vi "Teleop.vi"(10 "Match Info":T1={"Autonomous Elapsed Seconds"=0.0, "TeleOp Elapsed Seconds"=0.0, "Disabled Elapsed Seconds"=0.0, "Visited Autonomous"=FALSE, "Visited TeleOp"=FALSE, "Visited Disabled"=FALSE, "Autonomous Settings"={"Autonomous Style"=enum."Independent", "VI Refnum"=refnum}}, 11 "Call Context":T2) -> ()   [LabVIEW 2015]
doc: "This VI is called for each TeleOp packet received from the DS where the robot is not disabled. It is often used to read from the joysticks and update I/O or to update setpoints for timed control loops. It should complete and return within 20 milliseconds or it may miss DS packets."
uses:
  <vilib>/Rock Robotics/WPI/DriverStation/WPI_DriverStationDerivedRobotMode.ctl
  <vilib>/Rock Robotics/WPI/DriverStation/WPI_DriverStationMatch Info.ctl
  <vilib>/Rock Robotics/Network Tables/NT Read Boolean.vi
  <vilib>/Rock Robotics/Network Tables/NT Read Number.vi
  <vilib>/Rock Robotics/WPI/Utilities/WPI_GetSetVariantRefNum.vi
  <vilib>/Rock Robotics/WPI/RobotDrive/WPI_RobotDriveArcadeDrive_Standard(NoSaturation).vi
  <vilib>/Rock Robotics/Network Tables/NT Write Numeric Array.vi
  Mr. Thayer 2.0.vi
  Mr. Thayer.vi
  <vilib>/Rock Robotics/Network Tables/NT Write Boolean Array.vi
  Global 3.vi
  Global 4.vi
panel:
  out "Sample Slider 0":dbl(slide) scale=0.0..5.0
  out "Sample Boolean 1":bool
  out "Sample Boolean 0":bool
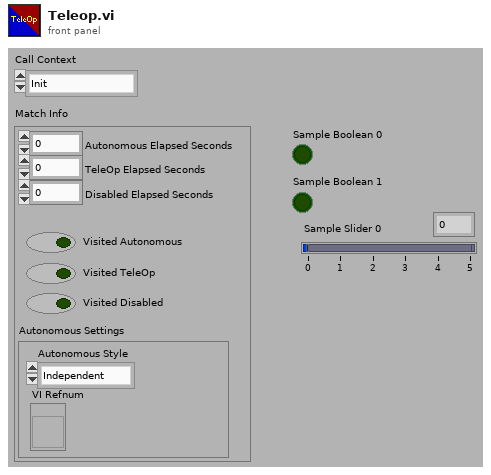
[diagram p1: front panel]
types:
  T1 = typedef "WPI_DriverStationMatch Info.ctl" = cluster{"Autonomous Elapsed Seconds":dbl, "TeleOp Elapsed Seconds":dbl, "Disabled Elapsed Seconds":dbl, "Visited Autonomous":bool, "Visited TeleOp":bool, "Visited Disabled":bool, "Autonomous Settings":cluster{"Autonomous Style":enum16{"Iterative", "Independent"}, "VI Refnum":refnum<vi>}}
  T2 = typedef "WPI_DriverStationDerivedRobotMode.ctl" = enum16{"Init", "Execute", "Stop"}
  T3 = typedef "WPI_JoystickDevRef.ctl" = cluster{"Device":T4}
  T4 = typedef "WPI_JoystickDeviceEnum.ctl" = enum16{"USB 0", "USB 1", "USB 2", "USB 3", "USB 4", "USB 5"}
  T5 = cluster{"Buttons[0]":bool, "Buttons[1]":bool, "Buttons[2]":bool, "Buttons[3]":bool, "Buttons[4]":bool, "Buttons[5]":bool, "Buttons[6]":bool, "Buttons[7]":bool, "Buttons[8]":bool}
  T6 = typedef "WPI_MotorControlDeviceRef.ctl" = cluster{"DeviceStatus":errorcluster, "Type":T7, "PWM":cluster{"PWM Channel":T8, "DeadBand":T9}, "CAN":cluster{"Device Number":u8, "Control Mode":T10, "Semaphore":T11, "Max Vout":dbl, "TalonSRX Control Mode":T12}, "Invert":bool}
  T7 = typedef "WPI_MotorControlType.ctl" = enum16{"PWM", "CAN", "CANTalonSRX"}
  T8 = typedef "FPGA_DIOPWMChannel.ctl" = enum8{"PWM 0", "PWM 1", "PWM 2", "PWM 3", "PWM 4", "PWM 5", "PWM 6", "PWM 7", "PWM 8", "PWM 9", "PWM MXP 0", "PWM MXP 1", "PWM MXP 2", "PWM MXP 3", "PWM MXP 4", "PWM MXP 5", "PWM MXP 6", "PWM MXP 7", "PWM MXP 8", "PWM MXP 9", "Invalid"}
  T9 = typedef "WPI_PWMDeadband.ctl" = cluster{"Name":string, "maxPositivePwm":i32, "minPositivePwm":i32, "centerPwm":i32, "maxNegativePwm":i32, "minNegativePwm":i32, "angularRange":u16}
  T10 = typedef "WPI_CANJaguar_ControlMode.ctl" = enum8{"Percent VBus", "Current", "Speed", "Position", "Voltage"}
  T11 = typedef "Semaphore RefNum" = refnum<k1>
  T12 = typedef "WPI_CANTalonSRX_APIControlMode.ctl" = enum8{"Percent VBus", "Speed", "Position", "Slave", "Unchanged / Invalid", "Voltage Compensation", "Current", "Motion Profile"}
  T13 = typedef "WPI_RobotDriveDevRef.ctl" = cluster{"DevStatus":errorcluster, "Motors[]":T6[], "Square Inputs":bool, "Max Output":dbl}
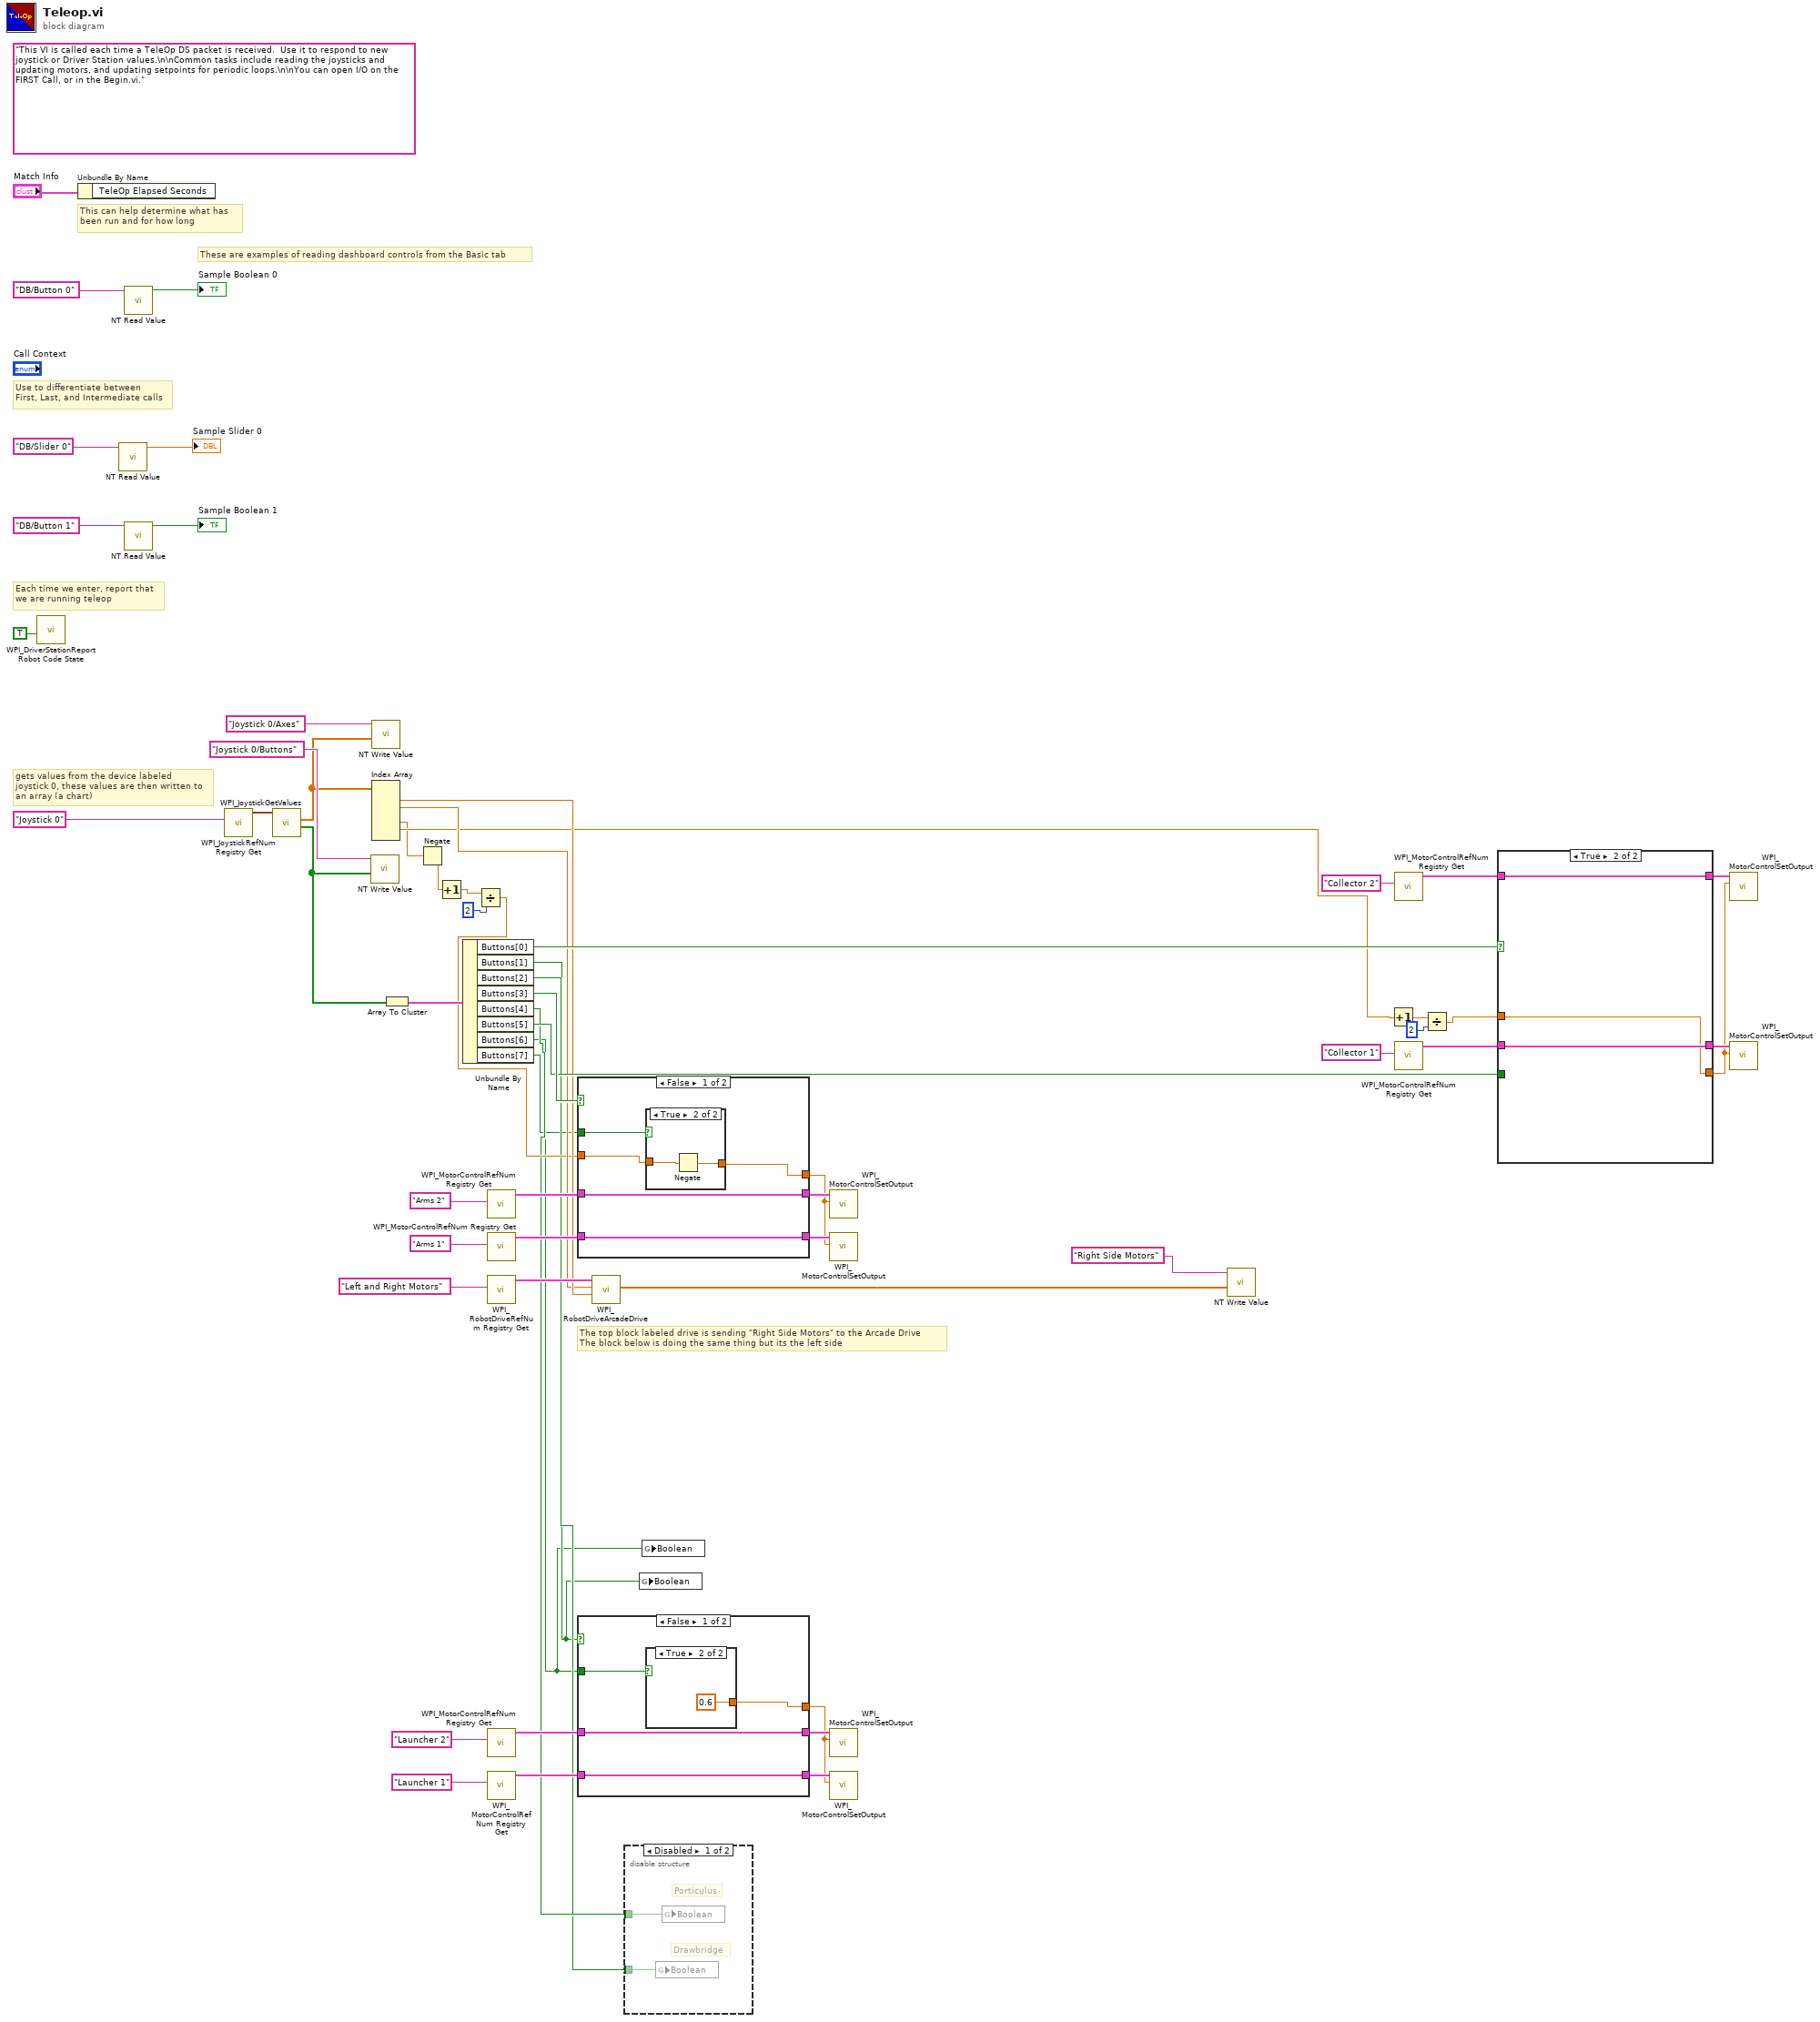
[diagram p0: block diagram]
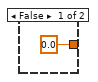
[diagram p3: hidden frame]
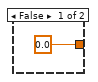
[diagram p5: hidden frame]
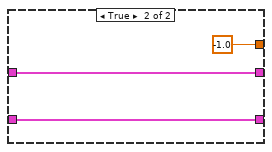
[diagram p6: hidden frame]
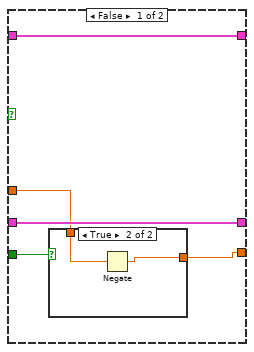
[diagram p7: hidden frame]
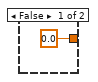
[diagram p8: hidden frame]
diagram:
  (unwired) "This VI is called each time a TeleOp DS packet is received.  Use it to respond to new joystick or Driver Station values.\n\nCommon tasks include reading the joysticks and updating motors, and updating setpoints for periodic loops.\n\nYou can open I/O on the FIRST Call, or in the Begin.vi."
  # "The top block labeled drive is sending \"Right Side Motors\" to the Arcade Drive \nThe block below is doing the same thing but its the left side"
  # "gets values from the device labeled \njoystick 0, these values are then written to\nan array (a chart)"
  # "These are examples of reading dashboard controls from the Basic tab"
  # "Each time we enter, report that\nwe are running teleop"
  # "Use to differentiate between\nFirst, Last, and Intermediate calls"
  # "This can help determine what has\nbeen run and for how long"
  n1 = call <vilib>:"WPI_DriverStationReport Robot Code State.vi"("TeleOp"=TRUE ("Autonomous")) -> ()  [unwired: 10 in, 1 out]
  n2 = Unbundle By Name("Match Info") -> ()  [unwired: 1 out]
  n3 = call-poly <vilib>:"NT Read Value.vi"("Name"="DB/Slider 0" ("refnum name")) -> ("Numeric"=→"Sample Slider 0":dbl)  [unwired: 9 in, 1 out]
  n4 = call-poly <vilib>:"NT Read Value.vi"("Name"="DB/Button 0" ("refnum name")) -> ("Boolean"=→"Sample Boolean 0":bool)  [unwired: 9 in, 1 out]
  n5 = call-poly <vilib>:"NT Read Value.vi"("Name"="DB/Button 1" ("refnum name")) -> ("Boolean"=→"Sample Boolean 1":bool)  [unwired: 9 in, 1 out]
  n6 = call <vilib>:"WPI_JoystickRefNum Registry Get.vi"("refnum name"="Joystick 0") -> ("JoystickDevRef"=w58:T3)  [unwired: 1 in, 9 out]
  n7 = call <vilib>:"WPI_JoystickGetValues.vi"("JoystickDevRef"=w58) -> ("Buttons"=w18:bool[], "Axes"=w55:dbl[])  [unwired: 6 in, 3 out]
  n8 = call-poly <vilib>:"NT Write Value.vi"("Boolean Array"=w18, "Name"="Joystick 0/Buttons") -> ()  [unwired: 9 in, 1 out]
  n9 = call-poly <vilib>:"NT Write Value.vi"("Numeric Array"=w55, "Name"="Joystick 0/Axes") -> ()  [unwired: 9 in, 1 out]
  n10 = Index Array(array=w55) -> (element #1=w16:dbl, element #2=w15:dbl, element #4=w4:dbl, element #5=w11:dbl)  [unwired: 6 in, 2 out]
  n11 = Array To Cluster(array=w18) -> (cluster=w48:T5)
  n12 = Negate(x=w4) -> (-x=w5:dbl)
  n13 = Increment(x=w5) -> (x+1=w14:dbl)
  n14 = Unbundle By Name(w48) -> ("Buttons[0]"=w41:bool, "Buttons[1]"=w2:bool, "Buttons[2]"=w6:bool, "Buttons[3]"=w47:bool, "Buttons[4]"=w7:bool, "Buttons[5]"=w17:bool, "Buttons[6]"=w1:bool, "Buttons[7]"=w3:bool)
  n15 = Divide(x=w14, y=2) -> (x/y=w12:dbl)
  n16 = call <vilib>:"WPI_MotorControlRefNum Registry Get.vi"("refnum name"="Arms 2") -> ("MotorControlDevRef"=w30:T6)  [unwired: 9 in, 1 out]
  n17 = call <vilib>:"WPI_MotorControlRefNum Registry Get.vi"("refnum name"="Arms 1") -> ("MotorControlDevRef"=w32:T6)  [unwired: 9 in, 1 out]
  n18 = call <vilib>:"WPI_RobotDriveRefNum Registry Get.vi"("refnum name"="Left and Right Motors") -> ("RobotDriveDevRef"=w45:T13)  [unwired: 9 in, 1 out]
  n19 = call <vilib>:"WPI_MotorControlRefNum Registry Get.vi"("refnum name"="Launcher 2") -> ("MotorControlDevRef"=w35:T6)  [unwired: 9 in, 1 out]
  n20 = call <vilib>:"WPI_MotorControlRefNum Registry Get.vi"("refnum name"="Launcher 1") -> ("MotorControlDevRef"=w37:T6)  [unwired: 9 in, 1 out]
  n21 = case shown="False" w47 {
    tunnel: [w64 w70] -> w33
    tunnel: w32 -> [w64 w70]
    tunnel: [w63 w69] -> w31
    tunnel: w30 -> [w63 w69]
    tunnel: [w62 w68] -> w27
    tunnel: w12 -> [w61 w68]
    tunnel: w3 -> [w60 _]
    frame False {
      n22 = case shown="True" w60 {
        tunnel: [0.0 w67] -> w62
        tunnel: w61 -> [_ w66]
        frame False {
        }
        frame True {
          n23 = Negate(x=w66) -> (-x=w67:dbl)
        }
      }
    }
    frame True {
    }
  }
  n24 = case shown="False" w2 {
    tunnel: [w74 w79] -> w38
    tunnel: w37 -> [w74 w79]
    tunnel: [w73 w78] -> w36
    tunnel: w35 -> [w73 w78]
    tunnel: [w72 -1.0] -> w34
    tunnel: w1 -> [w71 _]
    frame False {
      n25 = case shown="True" w71 {
        tunnel: [0.0 0.6] -> w72
        frame False {
        }
        frame True {
        }
      }
    }
    frame True {
    }
  }
  n26 = call-poly <vilib>:"WPI_RobotDriveArcadeDrive.vi"("Y axis value"=w16, "X axis value"=w15, "RobotDriveDevRef"=w45) -> ("Motor Values"=w44:dbl[])  [unwired: 6 in, 2 out]
  n27 = disable-structure shown="Disabled" {
    disable-tunnel: w7 -> [w81 _]
    disable-tunnel: w6 -> [w80 _]
    frame Disabled {
      # "Drawbridge"
      # "Porticulus"
      n28 = global write "Global 4.vi" "Boolean"(w80) -> ()
      n29 = global write "Global 3.vi" "Boolean"(w81) -> ()
    }
    frame Enabled {
    }
  }
  n30 = global write "Mr. Thayer.vi" "Boolean"(w2) -> ()
  n31 = global write "Mr. Thayer 2.0.vi" "Boolean"(w1) -> ()
  n32 = call <vilib>:"WPI_MotorControlSetOutput.vi"("Output"=w27, "MotorControlDevRef"=w31) -> ()  [unwired: 7 in, 3 out]
  n33 = call <vilib>:"WPI_MotorControlSetOutput.vi"("Output"=w27, "MotorControlDevRef"=w33) -> ()  [unwired: 7 in, 3 out]
  n34 = call <vilib>:"WPI_MotorControlSetOutput.vi"("Output"=w34, "MotorControlDevRef"=w36) -> ()  [unwired: 7 in, 3 out]
  n35 = call <vilib>:"WPI_MotorControlSetOutput.vi"("Output"=w34, "MotorControlDevRef"=w38) -> ()  [unwired: 7 in, 3 out]
  n36 = call-poly <vilib>:"NT Write Value.vi"("Numeric Array"=w44, "Name"="Right Side Motors") -> ()  [unwired: 9 in, 1 out]
  n37 = Increment(x=w11) -> (x+1=w10:dbl)
  n38 = call <vilib>:"WPI_MotorControlRefNum Registry Get.vi"("refnum name"="Collector 2") -> ("MotorControlDevRef"=w23:T6)  [unwired: 9 in, 1 out]
  n39 = call <vilib>:"WPI_MotorControlRefNum Registry Get.vi"("refnum name"="Collector 1") -> ("MotorControlDevRef"=w25:T6)  [unwired: 9 in, 1 out]
  n40 = Divide(x=w10, y=2) -> (x/y=w8:dbl)
  n41 = case shown="True" w41 {
    tunnel: [w85 w90] -> w22
    tunnel: [w86 w92] -> w26
    tunnel: w25 -> [w86 w92]
    tunnel: [w84 w91] -> w24
    tunnel: w23 -> [w84 w91]
    tunnel: w17 -> [w83 _]
    tunnel: w8 -> [w82 w90]
    frame False {
      n42 = case shown="True" w83 {
        tunnel: [0.0 w88] -> w85
        tunnel: w82 -> [_ w89]
        frame False {
        }
        frame True {
          n43 = Negate(x=w89) -> (-x=w88:dbl)
        }
      }
    }
    frame True {
    }
  }
  n44 = call <vilib>:"WPI_MotorControlSetOutput.vi"("Output"=w22, "MotorControlDevRef"=w24) -> ()  [unwired: 7 in, 3 out]
  n45 = call <vilib>:"WPI_MotorControlSetOutput.vi"("Output"=w22, "MotorControlDevRef"=w26) -> ()  [unwired: 7 in, 3 out]
